vi "GetFPNativeWind.vi"(0 "VI Ref In":refnum<vi>, 11 "Error In":errorcluster caption="entrée d'erreur (pas d'erreur)") -> (4 "VI Ref Out":refnum<vi>, 8 "Front Panel Window Handler":u64, 15 "Error Out":errorcluster caption="sortie d'erreur")   [LabVIEW 2020]
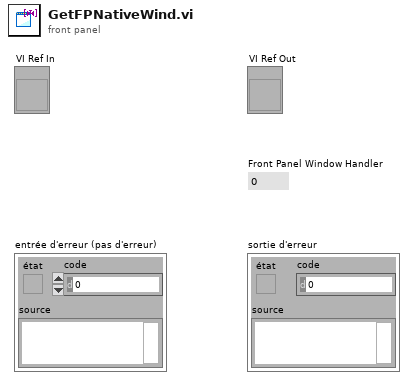
[diagram p1: front panel]
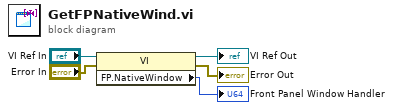
[diagram p0: block diagram]
diagram:
  n1 = property class="VI"(reference="VI Ref In", error in="Error In") -> (reference out=→"VI Ref Out":refnum<vi>, error out=→"Error Out":errorcluster, "FP.NativeWindow"=→"Front Panel Window Handler":u64)
